vi "(SubVI) XYZ information for Stage and DAQ channel_YCC.vi"(4 "Axis  (Enum)":enum16{"x", "y", "z"}(ring)) -> (1 "physical channels":tag, 2 "Axis":i32)   [LabVIEW 2014]
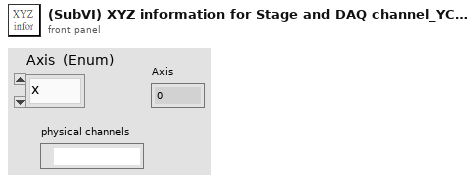
[diagram p1: front panel]
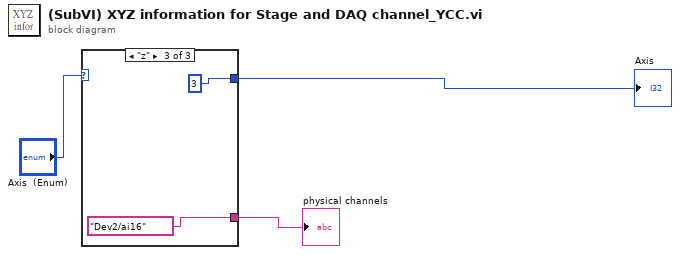
[diagram p0: block diagram]
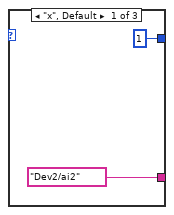
[diagram p2: hidden frame]
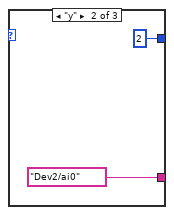
[diagram p3: hidden frame]
diagram:
  n1 = case shown="\"z\"" "Axis  (Enum)" {
    tunnel: [1 2 3] -> w2
    tunnel: [tag "Dev2/ai2" ("physical channels") tag "Dev2/ai0" ("physical channels") tag "Dev2/ai16" ("physical channels")] -> w3
    frame "x", Default {
    }
    frame "y" {
    }
    frame "z" {
    }
  }
  "physical channels" <- w3
  "Axis" <- w2
